vi "Select Controller Init Objects.vi"(7 "Initial Controller":refnum<class "Controller.lvclass">, 10 "Controller":refnum<class "Controller.lvclass">, 11 "Inputs":refnum<class "Processing.lvclass">) -> (3 "Updated Inputs":refnum<class "Processing.lvclass">, 5 "Trace Message":string)   [LabVIEW 2020, in "HTTP Server.lvlib" / "Server.lvclass"]
uses:
  Server.lvclass
  Server.lvclass/Server.ctl
  Controller/Controller.lvclass
  C:/dev/lv20CE/relink/lv-http-server/HTTP Server/Controller/Controller.lvclass
  C:/dev/lv20CE/relink/lv-http-server/HTTP Server/Handler/Handler.lvclass
  Processing/Processing.lvclass
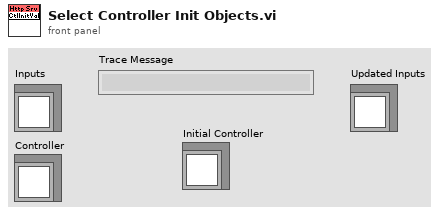
[diagram p1: front panel]
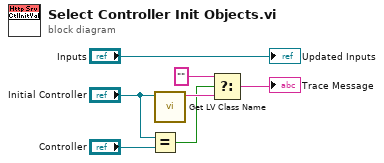
[diagram p0: block diagram]
diagram:
  n1 = Equal?(x="Initial Controller", y="Controller") -> (x = y?=w6:bool)
  n2 = call <vilib>:"Get LV Class Name.vi"("object"="Initial Controller") -> ("class name"=w7:string)  [unwired: 9 in, 1 out]
  n3 = Select(t="", s=w6, f=w7) -> (s? t:f=→"Trace Message":string)
  "Updated Inputs" <- "Inputs"
